vi "autopilot.vi"() -> ()   [LabVIEW 2015]
uses:
  global.vi
  <vilib>/addons/control/pid/pid.llb/PID (DBL).vi
  <vilib>/addons/control/pid/NI_PID_pid.lvlib
panel:
  out "Numeric 2":dbl
  out "Numeric":dbl
  in  "stop":bool
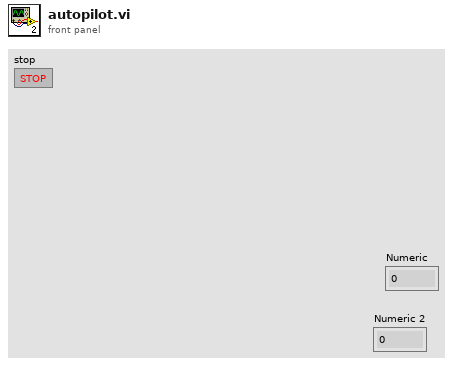
[diagram p1: front panel]
types:
  T1 = cluster{"Airspeed":dbl, "Altitude":dbl, "Vertical Speed":dbl, "Pitch":dbl, "Roll":dbl, "Heading":dbl, "Turn Indicator":dbl, "Latitude":dbl, "Longitude":dbl}
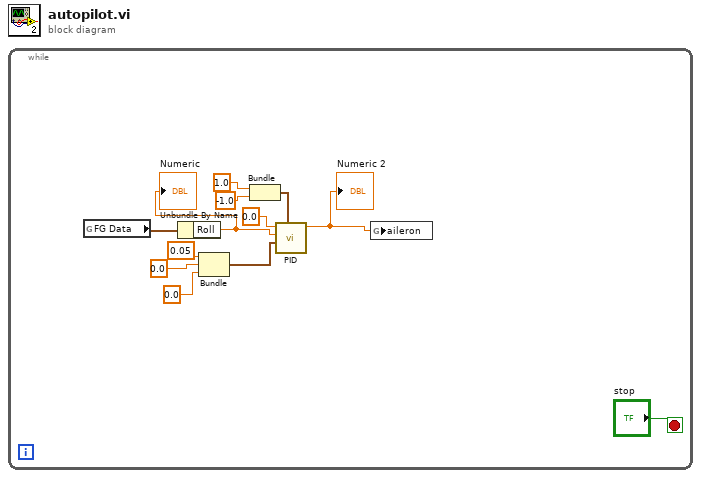
[diagram p0: block diagram]
diagram:
  n1 = while {
    stop <- "stop" stop-if-true
    n2 = global read "global.vi" "FG Data"() -> (w1:T1)
    n3 = Unbundle By Name(w1) -> ("Roll"=w10:dbl)
    "Numeric" <- w10
    n4 = Bundle(0.05, 0.0, 0.0) -> (w7:cluster{dbl, dbl, dbl})  [unwired: 1 in]
    n5 = Bundle(1.0, -1.0) -> (w4:cluster{dbl, dbl})  [unwired: 1 in]
    n6 = call-poly <vilib>:"PID.vi"("output range"=w4, "PID gains"=w7, "process variable"=w10, "setpoint"=0.0) -> ("output"=w11:dbl)  [unwired: 6 in, 1 out]
    "Numeric 2" <- w11
    n7 = global write "global.vi" "aileron"(w11) -> ()
  }
